vi "PlantUpdate.vi"(10 "u":dbl, 11 "Plant":T2) -> (2 "X":T1, 3 "y":dbl)   [LabVIEW 2017]
uses:
  <vilib>/Analysis/Matrix/Datatypes/RealMatrix.ctl
  <vilib>/Analysis/Matrix/Numeric/Multiply/Multiply - R,RM.vi
  <vilib>/Analysis/Matrix/Numeric/Multiply/Multiply - RM,RM.vi
  <vilib>/Analysis/Matrix/Numeric/Add/Add - RM,RM.vi
  <vilib>/Analysis/Matrix/NI_Matrix.lvlib
panel:
  in  "Reinitialize":bool
  out "Y":T1
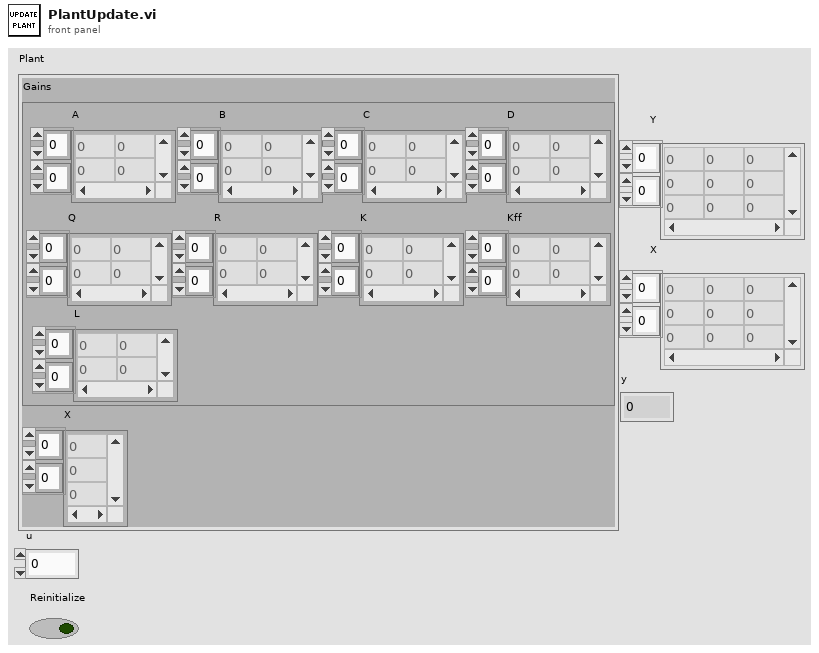
[diagram p1: front panel]
types:
  T1 = typedef "NI_Matrix.lvlib/RealMatrix.ctl" = dbl[][]
  T2 = cluster{"Gains":cluster{"A":T1, "B":T1, "C":T1, "D":T1, "Q":T1, "R":T1, "K":T1, "Kff":T1, "L":T1}, "X":T1}
  T3 = cluster{"A":T1, "B":T1, "C":T1, "D":T1, "Q":T1, "R":T1, "K":T1, "Kff":T1, "L":T1}
  T4 = cluster{"Gains":cluster{"A":T1, "B":T1, "C":T1, "D":T1, "Q":T1, "R":T1, "K":T1, "Kff":T1, "L":T1}, "A + B":T1}
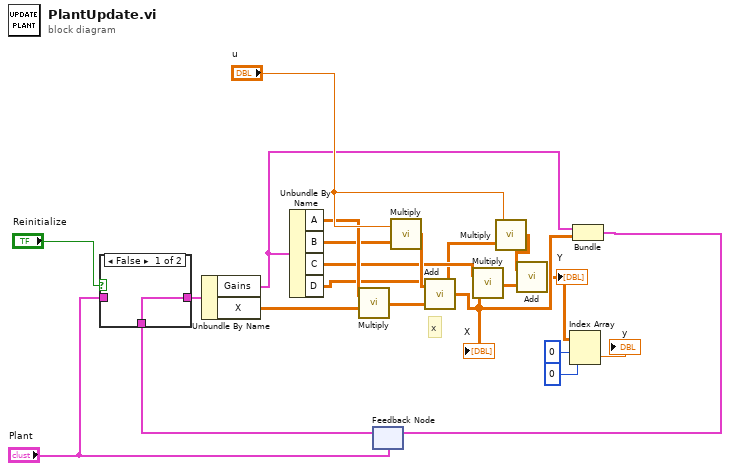
[diagram p0: block diagram]
diagram:
  # "x"
  n1 = feedback #1("Plant") -> (w4:T2)
  n2 = case shown="False" "Reinitialize" {
    tunnel: w4 -> [w22 _]
    tunnel: [w22 w23] -> w2
    tunnel: "Plant" -> [_ w23]
    frame False {
    }
    frame True {
    }
  }
  n3 = Unbundle By Name(w2) -> ("Gains"=w10:T3, "X"=w19:T1)
  n4 = Unbundle By Name(w10) -> ("A"=w18:T1, "B"=w16:T1, "C"=w14:T1, "D"=w12:T1)
  n5 = call-poly <vilib>:"Multiply.vi"("Real Matrix B"=w19, "Real Matrix A"=w18) -> ("A * B"=w17:T1)
  n6 = call-poly <vilib>:"Multiply.vi"("Real Matrix A"=w16, "Real Scalar c"="u") -> ("c * A"=w15:T1)
  n7 = call-poly <vilib>:"Add.vi"("Real Matrix B"=w17, "Real Matrix A"=w15) -> ("A + B"=w9:T1)
  "X" <- w9
  n8 = call-poly <vilib>:"Multiply.vi"("Real Matrix B"=w9, "Real Matrix A"=w14) -> ("A * B"=w13:T1)
  n9 = call-poly <vilib>:"Multiply.vi"("Real Matrix A"=w12, "Real Scalar c"="u") -> ("c * A"=w11:T1)
  n10 = call-poly <vilib>:"Add.vi"("Real Matrix B"=w13, "Real Matrix A"=w11) -> ("A + B"=w8:T1)
  "Y" <- w8
  n11 = Index Array(array=w8, index (row)=0, index (col)=0) -> (element=→"y":dbl)
  n12 = Bundle("Gains"=w10, "A + B"=w9) -> (w20:T4)  [unwired: 1 in]
  n13 = feedback-in #1(w20) -> ()
